vi "rszvl Initialize.vi"(0 "VISA resource name":refnum<visa-resource-name>, 5 "ID Query (T: Check)":bool=TRUE, 7 "Reset (T: Reset)":bool=TRUE, 11 "error in (no error)":errorcluster) -> (4 "VISA resource name out":refnum<visa-resource-name>, 15 "error out":errorcluster)   [LabVIEW 2014]
doc: "This VI open a new connection to the instrument.\nOptionally, you can reset the instrument.\nSetting *IDN? query to False will skip checking of the supported driver's instrument types.\nYou must run this VI or <b>Initialize with Options.vi</b> before using any of the instrument driver VIs."
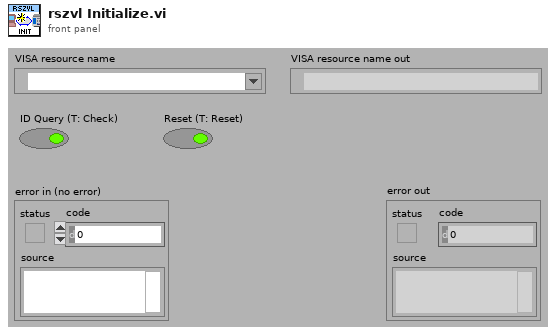
[diagram p1: front panel]
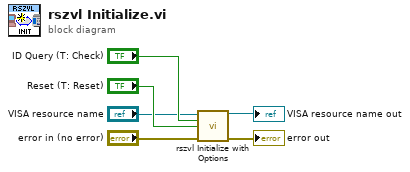
[diagram p0: block diagram]
diagram:
  n1 = call "rszvl Initialize with Options.vi"("VISA resource name"="VISA resource name", "ID Query (T: Check)"="ID Query (T: Check)", "Reset (T: Reset)"="Reset (T: Reset)", "error in (no error)"="error in (no error)") -> ("VISA resource name out"=→"VISA resource name out":refnum<visa-resource-name>, "error out"=→"error out":errorcluster)  [unwired: 10 in]
